vi "test move creation.vi"() -> ()   [LabVIEW 2016]
uses:
  Position/Position.lvclass
  Moves/Move/Move.lvclass
panel:
  out "Array 2":string[](array[string])
  out "Array":string[](array[string])
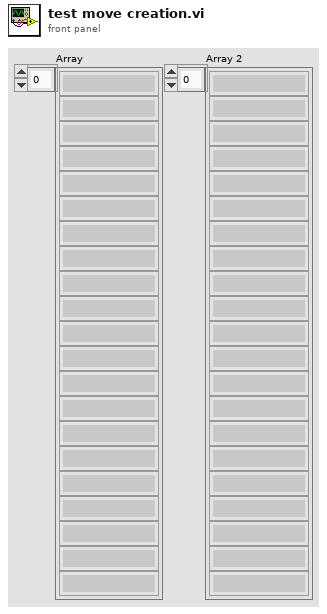
[diagram p1: front panel]
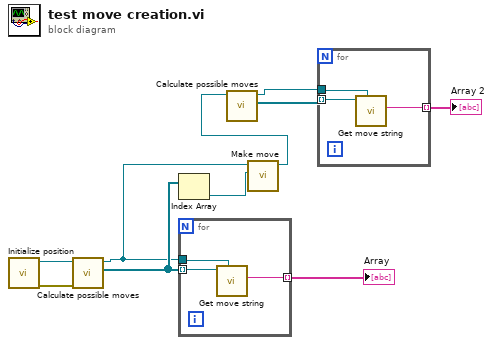
[diagram p0: block diagram]
diagram:
  n1 = call "Initialize position.vi"() -> ("error out"=w9:errorcluster, "Position out"=w10:refnum<class "Position.lvclass">)  [unwired: 10 in]
  n2 = call "Calculate possible moves.vi"("error in (no error)"=w9, "Position in"=w10) -> ("Moves"=w4:refnum<class "Move.lvclass">[], "Position out"=w2:refnum<class "Position.lvclass">)  [unwired: 7 in, 1 out]
  n3 = Index Array(array=w4) -> (element=w3:refnum<class "Move.lvclass">)  [unwired: 1 in]
  n4 = for {
    tunnel: w4 -> [w13] mode=indexing
    tunnel: [w12] -> w8 mode=indexing
    tunnel: w2 -> [w11]
    n5 = call "Get move string.vi"("Position"=w11, "Move in"=w13) -> ("Move string"=w12:string)  [unwired: 7 in, 2 out]
  }
  "Array" <- w8
  n6 = call "Make move.vi"("Move"=w3, "Position in"=w2) -> ("Position out"=w1:refnum<class "Position.lvclass">)  [unwired: 8 in, 1 out]
  n7 = call "Calculate possible moves.vi"("Position in"=w1) -> ("Moves"=w7:refnum<class "Move.lvclass">[], "Position out"=w6:refnum<class "Position.lvclass">)  [unwired: 8 in, 1 out]
  n8 = for {
    tunnel: w7 -> [w16] mode=indexing
    tunnel: [w15] -> w5 mode=indexing
    tunnel: w6 -> [w14]
    n9 = call "Get move string.vi"("Position"=w14, "Move in"=w16) -> ("Move string"=w15:string)  [unwired: 7 in, 2 out]
  }
  "Array 2" <- w5
